vi "picoharp_acquire_fast.vi"(8 "error in (no error)":errorcluster, 11 "hydraharp in":refnum<class "picoharp.lvclass">) -> (0 "error out":errorcluster, 3 "hydraharp out":refnum<class "picoharp.lvclass">)   [LabVIEW 2015, in "picoharp.lvclass"]
uses:
  picoharp.lvclass
  picoharp.lvclass/picoharp.ctl
  Hydraharp/hydraharp/hydraharp_fifo_queue_data.ctl
  Hydraharp/hydraharp/hydraharp_fifo_actions.ctl
  stop_pico_acq.vi
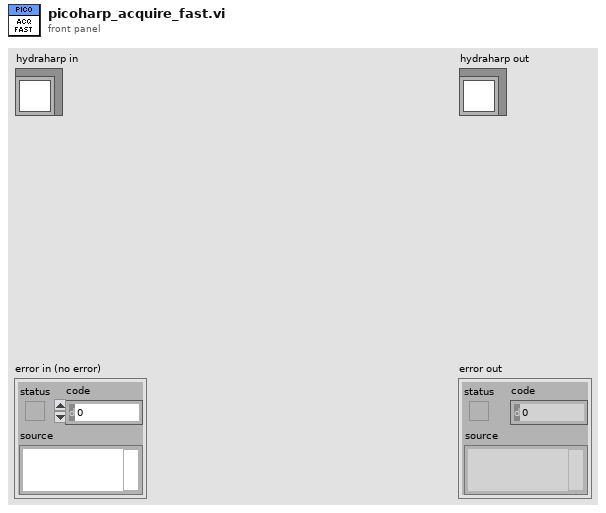
[diagram p1: front panel]
types:
  T1 = typedef "hydraharp_fifo_queue_data.ctl" = cluster{"fifo_buffer":u32[], "fifo_action":T2}
  T2 = typedef "hydraharp_fifo_actions.ctl" = enum16{"stop", "new_data"}
  T3 = cluster{"stop_fifo_stream":refnum<event-registration>, "Event Registration Refnum":refnum<event-registration>}
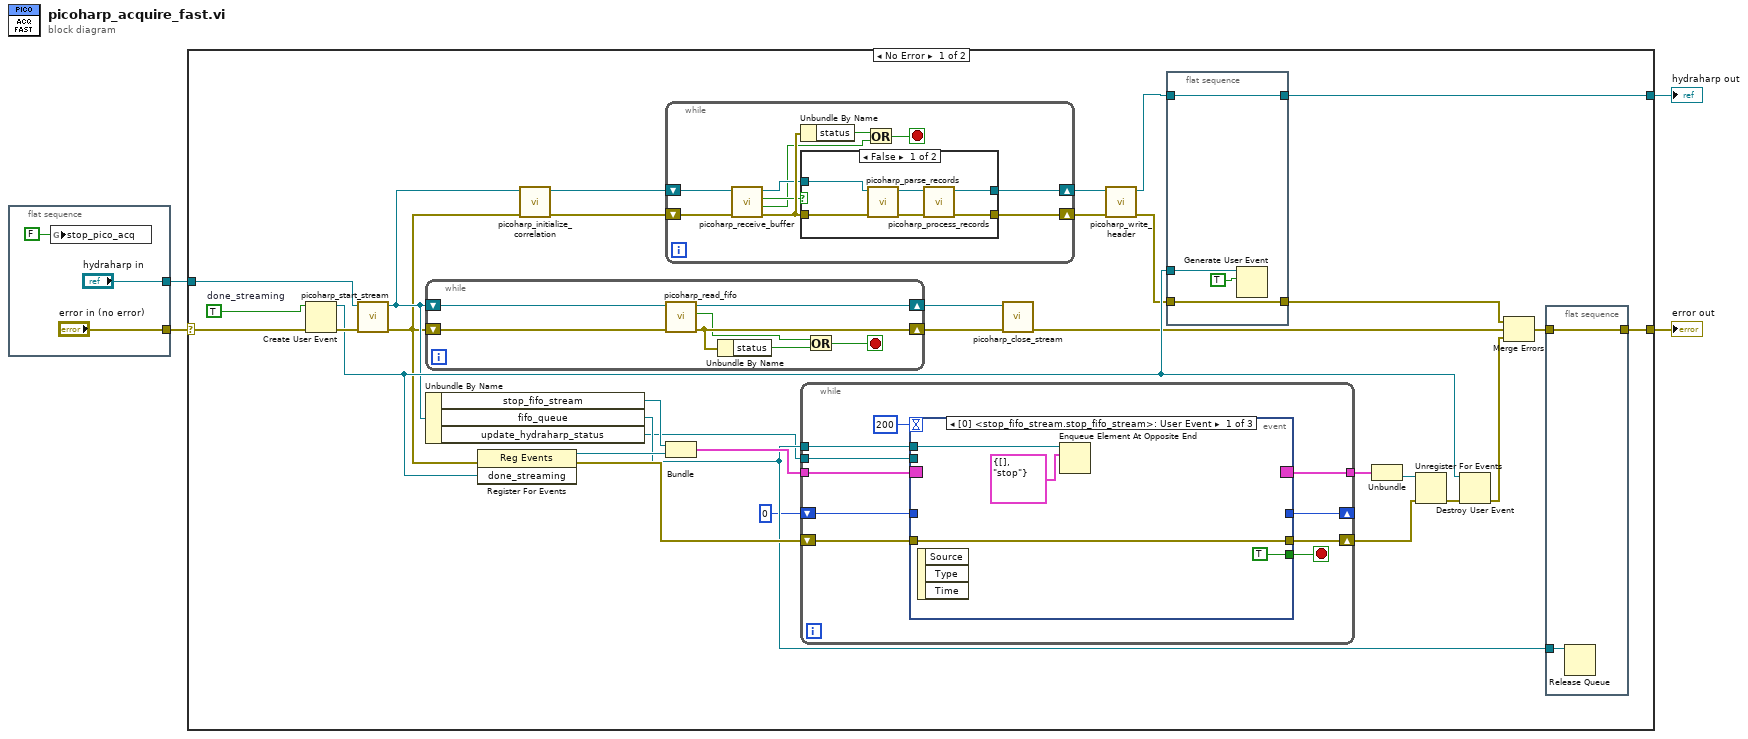
[diagram p0: block diagram]
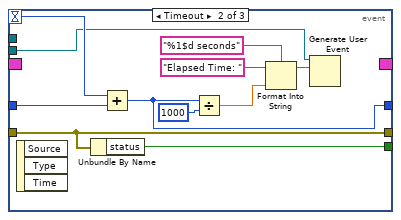
[diagram p2: hidden frame]
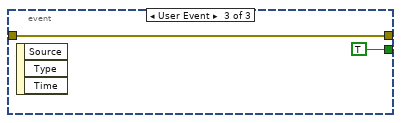
[diagram p3: hidden frame]
diagram:
  n1 = flat-sequence {
    tunnel: ["error in (no error)"] -> w4
    tunnel: ["hydraharp in"] -> w1
    frame #0 {
      n2 = global write "stop_pico_acq.vi" "stop_pico_acq"(FALSE ("stop_pico_acq")) -> ()
    }
  }
  n3 = case shown="No Error" w4 {
    selector: w4 -> [w38 w99]
    tunnel: [w37 w99] -> w3
    tunnel: [w36 w98] -> w2
    tunnel: w1 -> [w39 w98]
    frame No Error {
      w34 = TRUE  # done_streaming
      n4 = Create User Event(user event datatype=w34, error in=w38) -> (user event=w25:refnum<user-event>, error out=w32:errorcluster)
      n5 = call "picoharp_start_stream.vi"("error in (no error)"=w32, "hydraharp in"=w39) -> ("error out"=w18:errorcluster, "hydraharp out"=w20:refnum<class "picoharp.lvclass">)  [unwired: 8 in]
      n6 = while {
        shift-right: [w76] -> w11
        shift-left: w20 -> [w79]
        shift-right: [w77] -> w10
        shift-left: w18 -> [w78]
        stop <- w75 stop-if-true
        n7 = call "picoharp_read_fifo.vi"("error in (no error)"=w78, "hydraharp in"=w79) -> ("error out"=w77:errorcluster, "stop"=w73:bool, "hydraharp out"=w76:refnum<class "picoharp.lvclass">)  [unwired: 7 in]
        n8 = Unbundle By Name(w77) -> ("status"=w74:bool)
        n9 = Or(x=w73, y=w74) -> (x .or. y?=w75:bool)
      }
      n10 = Unbundle By Name(w20) -> ("stop_fifo_stream"=w31:refnum<event-registration>, "fifo_queue"=w21:refnum<queue>, "update_hydraharp_status"=w13:refnum<user-event>)
      n11 = register-events(error in=w18, w25) -> (reference out=w30:refnum<event-registration>, error out=w33:errorcluster)  [unwired: 1 in]
      n12 = call "picoharp_initialize_correlation.vi"("error in (no error)"=w18, "hydraharp in"=w20) -> ("error out"=w17:errorcluster, "hydraharp out"=w19:refnum<class "picoharp.lvclass">)  [unwired: 8 in]
      n13 = while {
        shift-right: [w83] -> w15
        shift-left: w19 -> [w88]
        shift-right: [w82] -> w16
        shift-left: w17 -> [w89]
        stop <- w86 stop-if-true
        n14 = call "picoharp_receive_buffer.vi"("error in (no error)"=w89, "hydraharp in"=w88) -> ("error out"=w85:errorcluster, "stop"=w80:bool, "queue_timed_out"=w81:bool, "hydraharp out"=w84:refnum<class "picoharp.lvclass">)  [unwired: 6 in]
        n15 = Unbundle By Name(w85) -> ("status"=w87:bool)
        n16 = case shown="False" w81 {
          tunnel: w85 -> [w92 w97]
          tunnel: w84 -> [w93 w96]
          tunnel: [w95 w96] -> w83
          tunnel: [w94 w97] -> w82
          frame False {
            n17 = call "picoharp_parse_records.vi"("error in (no error)"=w92, "hydraharp in"=w93) -> ("error out"=w90:errorcluster, "hydraharp out"=w91:refnum<class "picoharp.lvclass">)  [unwired: 8 in]
            n18 = call "picoharp_process_records.vi"("error in (no error)"=w90, "hydraharp in"=w91) -> ("error out"=w94:errorcluster, "hydraharp out"=w95:refnum<class "picoharp.lvclass">)  [unwired: 8 in]
          }
          frame True {
          }
        }
        n19 = Or(x=w87, y=w80) -> (x .or. y?=w86:bool)
      }
      n20 = Bundle("stop_fifo_stream"=w31, "Event Registration Refnum"=w30) -> (w29:T3)  [unwired: 1 in]
      n21 = while {
        tunnel: w21 -> [w54]
        tunnel: [w53] -> w28
        shift-right: [w50] -> w35
        shift-left: w33 -> [w51]
        tunnel: w29 -> [w49]
        shift-right: [w47] -> _
        shift-left: 0 -> [w48]
        tunnel: w13 -> [w46]
        stop <- w55 stop-if-true
        n22 = event shown="[0] <stop_fifo_stream.stop_fifo_stream>: User Event" {
          selector: w49 -> [_ _ _]
          dyn-events: [_ _ _] -> w53
          timeout: 200 -> [_ w63 _]
          tunnel: [TRUE w70 TRUE] -> w55
          tunnel: w54 -> [w58 _ _]
          tunnel: w51 -> [w56 w69 w71]
          tunnel: [w56 w69 w71] -> w50
          tunnel: w48 -> [_ w62 _]
          tunnel: [_ w61 _] -> w47
          tunnel: w46 -> [_ w60 _]
          event User Event {
            n23 = event-data() -> ()  [unwired: 1 in, 3 out]
            n24 = Enqueue Element At Opposite End(queue=w58, element=T1 {"fifo_buffer"=[], "fifo_action"=enum."stop"}) -> ()  [unwired: 2 in, 3 out]
          }
          event Timeout {
            n25 = event-data() -> ()  [unwired: 1 in, 3 out]
            n26 = Unbundle By Name(w69) -> ("status"=w70:bool)
            n27 = Add(x=w63, y=w62) -> (x+y=w61:i32)
            n28 = Divide(x=w61, y=1000) -> (x/y=w65:dbl)
            n29 = Format Into String(format string="%1$d seconds", initial string="Elapsed Time: ", w65) -> (resulting string=w64:string)  [unwired: 1 in, 1 out]
            n30 = Generate User Event(user event=w60, event data cluster=w64) -> ()  [unwired: 2 in, 2 out]
          }
          event User Event {
            n31 = event-data() -> ()  [unwired: 1 in, 3 out]
          }
        }
      }
      n32 = call "picoharp_close_stream.vi"("error in (no error)"=w10, "hydraharp in"=w11) -> ("error out"=w9:errorcluster)  [unwired: 8 in, 1 out]
      n33 = call "picoharp_write_header.vi"("error in (no error)"=w16, "hydraharp in"=w15) -> ("error out"=w12:errorcluster, "hydraharp out"=w8:refnum<class "picoharp.lvclass">)  [unwired: 8 in]
      n34 = flat-sequence {
        tunnel: w12 -> [w42]
        tunnel: w8 -> [w45]
        tunnel: [w45] -> w36
        tunnel: w25 -> [w44]
        tunnel: [w42] -> w24
        frame #0 {
          n35 = Generate User Event(user event=w44, event data cluster=TRUE ("event data")) -> ()  [unwired: 2 in, 2 out]
        }
      }
      n36 = Unbundle(w28) -> ("Event Registration Refnum"=w27:refnum<event-registration>)  [unwired: 1 out]
      n37 = Unregister For Events(event registration refnum=w27, error in=w35) -> (error out=w23:errorcluster)
      n38 = Destroy User Event(user event=w25, error in=w23) -> (error out=w26:errorcluster)
      n39 = Merge Errors(w24, w9, w26) -> (w22:errorcluster)
      n40 = flat-sequence {
        tunnel: w22 -> [w40]
        tunnel: w21 -> [w41]
        tunnel: [w40] -> w37
        frame #0 {
          n41 = Release Queue(queue=w41) -> ()  [unwired: 2 in, 3 out]
        }
      }
    }
    frame Error {
    }
  }
  "error out" <- w3
  "hydraharp out" <- w2
